vi "WAM_ESS.vi"(0 "VISA resource name":refnum<visa-resource-name>="COM5", 11 "error in (no error)":errorcluster, 12 "Open Serial":bool, 13 "Test Running (T)":bool, 14 "Close Serial":bool) -> (1 "Enabled(T-RO)":bool, 3 "FH_NOT(T)":bool, 4 "VISA resource name out":refnum<visa-resource-name>, 15 "error out":errorcluster)   [LabVIEW 2018]
panel:
  out "number":u32
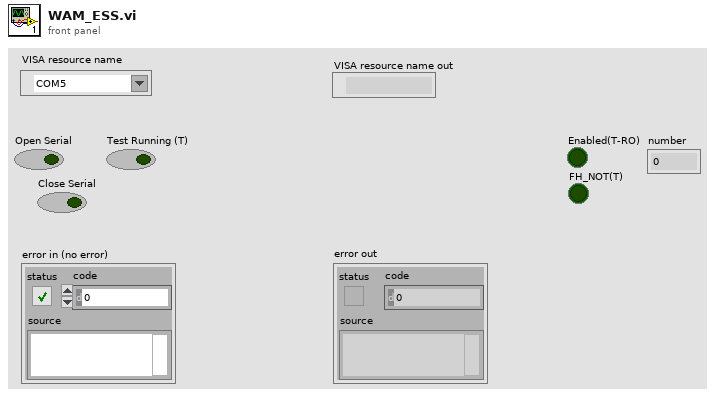
[diagram p1: front panel]
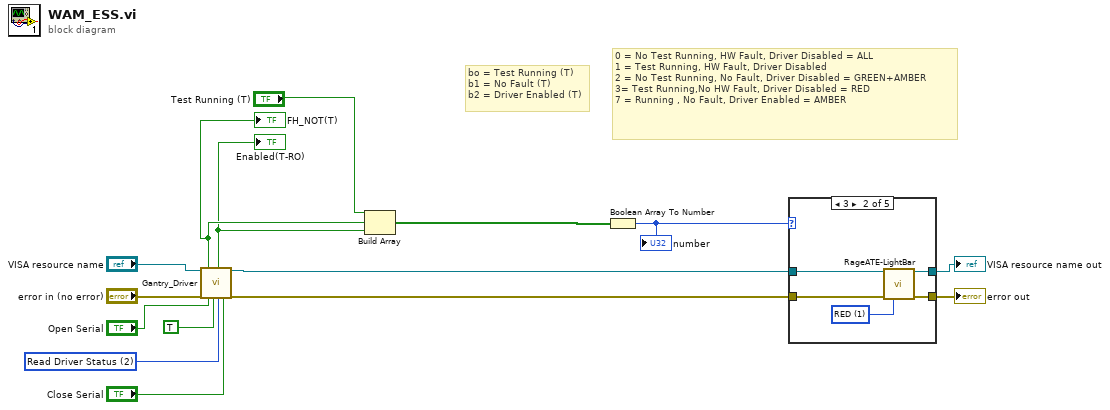
[diagram p0: block diagram]
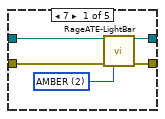
[diagram p2: hidden frame]
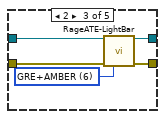
[diagram p3: hidden frame]
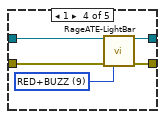
[diagram p4: hidden frame]
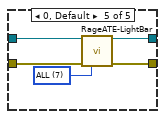
[diagram p5: hidden frame]
diagram:
  w7 = u16 2 items=["Disable Driver", "Enable Driver", "Read Driver Status"] ("Driver-Func")
  # "0 = No Test Running, HW Fault, Driver Disabled = ALL\n1 = Test Running, HW Fault, Driver Disabled\n2 = No Test Running, No Fault, Driver Disabled = GREEN+AMBER\n3= Test Running,No HW Fault, Driver Disabled = RED\n7 = Running , No Fault, Driver Enabled = AMBER"
  # "bo = Test Running (T) \nb1 = No Fault (T)\nb2 = Driver Enabled (T)"
  n1 = call "Gantry_Driver.vi"("VISA resource name"="VISA resource name", "error in (no error)"="error in (no error)", "Open Serial"="Open Serial", "RO(T)"=TRUE, "Driver-Func"=w7, "Close Serial"="Close Serial") -> ("FH_NOT(T)"=w4:bool, "Enabled(T-RO)"=w3:bool, "VISA resource name out"=w10:refnum<visa-resource-name>, "error out"=w11:errorcluster)  [unwired: 10 in]
  "Enabled(T-RO)" <- w3
  "FH_NOT(T)" <- w4
  n2 = Build Array("Test Running (T)", w4, w3) -> (w2:bool[])
  n3 = Boolean Array To Number(Boolean array=w2) -> (number=w1:u32)
  "number" <- w1
  n4 = case shown="3" w1 {
    tunnel: [w20 w25 w30 w35 w40] -> w13
    tunnel: [w19 w24 w29 w34 w39] -> w12
    tunnel: w11 -> [w18 w23 w28 w33 w38]
    tunnel: w10 -> [w17 w22 w27 w32 w37]
    frame 7 {
      w16 = u32 2 items=["OFF"=0, "RED"=1, "AMBER"=2, "GREEN"=4, "ALL"=7, "BUZZ"=8, "RED+BUZZ"=9, "ALL+BUZZ"=15] ("Select")
      n5 = call "RageATE-LightBar.vi"("VISA resource name"=w17, "error in"=w18, "Select"=w16) -> ("VISA resource name out"=w19:refnum<visa-resource-name>, "error out"=w20:errorcluster)  [unwired: 10 in, 1 out]
    }
    frame 3 {
      w21 = u32 1 items=["OFF"=0, "RED"=1, "AMBER"=2, "GREEN"=4, "ALL"=7, "BUZZ"=8, "RED+BUZZ"=9, "ALL+BUZZ"=15] ("Select")
      n6 = call "RageATE-LightBar.vi"("VISA resource name"=w22, "error in"=w23, "Select"=w21) -> ("VISA resource name out"=w24:refnum<visa-resource-name>, "error out"=w25:errorcluster)  [unwired: 10 in, 1 out]
    }
    frame 2 {
      w26 = u32 6 items=["OFF"=0, "RED"=1, "AMBER"=2, "GREEN"=4, "GRE+AMBER"=6, "ALL"=7, "BUZZ"=8, "RED+BUZZ"=9, "ALL+BUZZ"=15] ("Select")
      n7 = call "RageATE-LightBar.vi"("VISA resource name"=w27, "error in"=w28, "Select"=w26) -> ("VISA resource name out"=w29:refnum<visa-resource-name>, "error out"=w30:errorcluster)  [unwired: 10 in, 1 out]
    }
    frame 1 {
      w31 = u32 9 items=["OFF"=0, "RED"=1, "AMBER"=2, "GREEN"=4, "ALL"=7, "BUZZ"=8, "RED+BUZZ"=9, "ALL+BUZZ"=15] ("Select")
      n8 = call "RageATE-LightBar.vi"("VISA resource name"=w32, "error in"=w33, "Select"=w31) -> ("VISA resource name out"=w34:refnum<visa-resource-name>, "error out"=w35:errorcluster)  [unwired: 10 in, 1 out]
    }
    frame 0, Default {
      w36 = u32 7 items=["OFF"=0, "RED"=1, "AMBER"=2, "GREEN"=4, "ALL"=7, "BUZZ"=8, "RED+BUZZ"=9, "ALL+BUZZ"=15] ("Select")
      n9 = call "RageATE-LightBar.vi"("VISA resource name"=w37, "error in"=w38, "Select"=w36) -> ("VISA resource name out"=w39:refnum<visa-resource-name>, "error out"=w40:errorcluster)  [unwired: 10 in, 1 out]
    }
  }
  "error out" <- w13
  "VISA resource name out" <- w12
